vi "Start.vi"(8 "error in (no error)":errorcluster, 11 "Electrophysiology in":refnum<class "BehaviorData.lvclass">) -> (0 "error out":errorcluster, 3 "Electrophysiology out":refnum<class "BehaviorData.lvclass">)   [LabVIEW 2014, in "BehaviorData.lvclass"]
uses:
  BehaviorData.lvclass
  BehaviorData.lvclass/BehaviorData.ctl
  AcquireTraces/AcquireTraces.lvclass
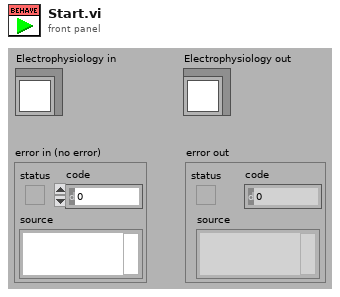
[diagram p1: front panel]
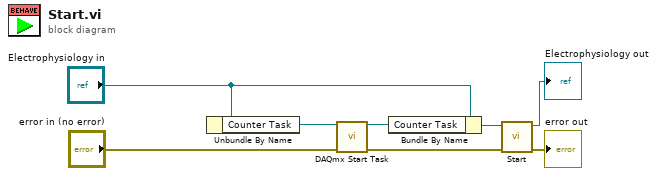
[diagram p0: block diagram]
diagram:
  n1 = Unbundle By Name("Electrophysiology in") -> ("Counter Task"=w2:refnum<k21>)
  n2 = call <vilib>:"DAQmx Start Task.vi"("task/channels in"=w2, "error in"="error in (no error)") -> ("task out"=w5:refnum<k21>, "error out"=w4:errorcluster)  [unwired: 12 in]
  n3 = Bundle By Name(cluster="Electrophysiology in", "Counter Task"=w5) -> (w6:refnum<class "BehaviorData.lvclass">)
  n4 = call-parent "Start.vi"("error in (no error)"=w4, "Electrophysiology in"=w6) -> ("error out"=→"error out":errorcluster, "Electrophysiology out"=→"Electrophysiology out":refnum<class "BehaviorData.lvclass">)  [unwired: 8 in]
